vi "SetDA.vi"() -> ()   [LabVIEW 2014]
uses:
  ESLSCDLL.dll
panel:
  in  "gain for TI amp":u8
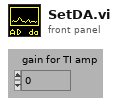
[diagram p1: front panel]
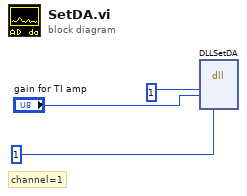
[diagram p0: block diagram]
diagram:
  # "channel=1"
  n1 = dll-call lib="C:/Users/Gerhard/Documents/New64/lv/1cam/board.vis/ESLSCDLL.dll" fn="DLLSetDA"("drv"=u32 1, "gain"="gain for TI amp", "ch"=u8 1) -> ()  [unwired: 7 in, 2 out]
